vi "Fixated Autoadjust.vi"(10 "Input":variant, 11 "Data":T1) -> (2 "Fixated":bool, 3 "Adjustment":dbl[](array[numeric]))   [LabVIEW 2010]
uses:
  Core SubVIs/Controls/TYPE - Analog Data.ctl
  <vilib>/Analysis/baseanly.llb/Unimode.vi
  <vilib>/Analysis/NI_AALBase.lvlib
  Core SubVIs/Core SubVIs.lvlib
panel:
  out "Max. running window size":i32=1000
  in  "Learning rate":dbl=0.0003
  in  "Minimum for update":i32=40
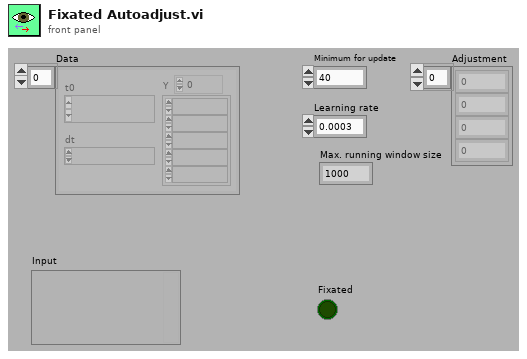
[diagram p1: front panel]
types:
  T1 = typedef "Core SubVIs.lvlib/TYPE - Analog Data.ctl" = waveform(dbl)[]
  T2 = cluster{"Trial Type":dbl, "Joystick Threshold":dbl, "Fixation Radius":dbl}
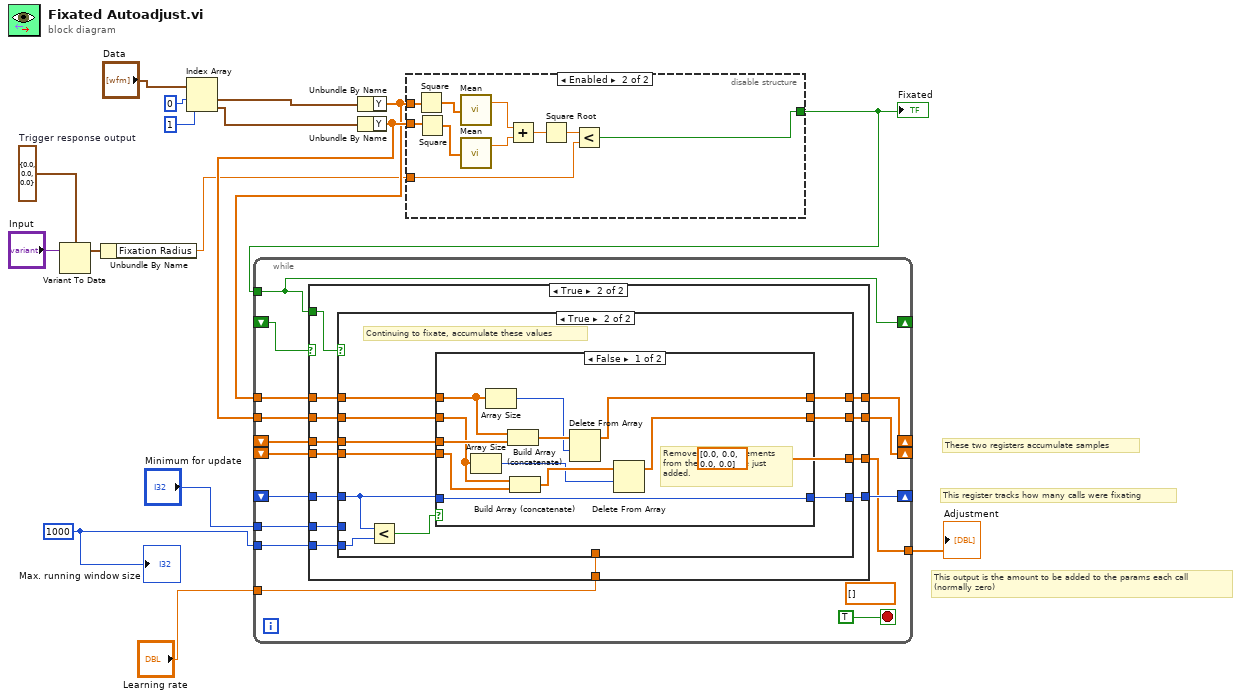
[diagram p0: block diagram]
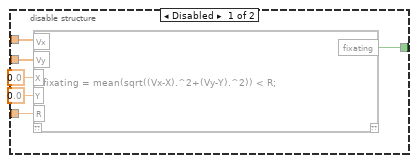
[diagram p2: hidden frame]
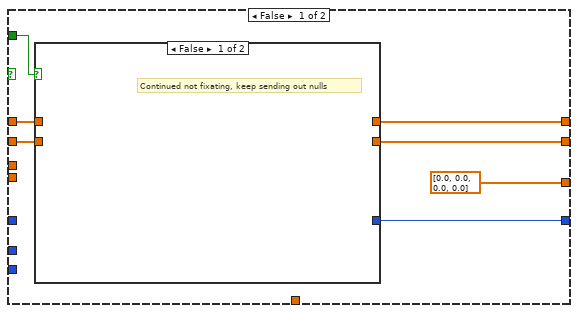
[diagram p3: hidden frame]
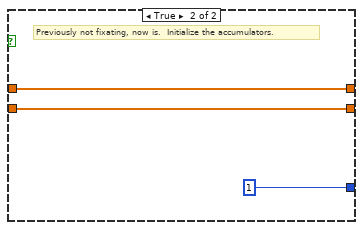
[diagram p4: hidden frame]
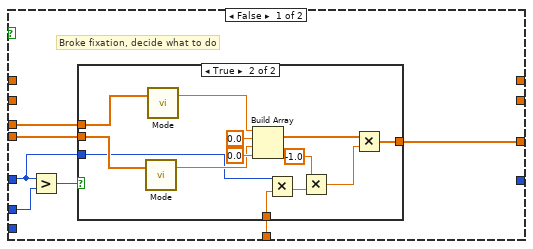
[diagram p5: hidden frame]
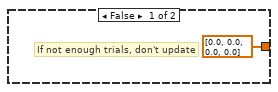
[diagram p6: hidden frame]
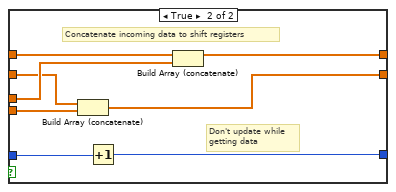
[diagram p7: hidden frame]
diagram:
  w3 = T2 {"Trial Type"=0.0, "Joystick Threshold"=0.0, "Fixation Radius"=0.0}  # Trigger response output
  w5 = 1000
  # "This output is the amount to be added to the params each call\n(normally zero)"
  # "These two registers accumulate samples"
  # "This register tracks how many calls were fixating"
  n1 = Variant To Data(Variant="Input", type=w3) -> (data=w2:T2)  [unwired: 1 in, 1 out]
  n2 = Unbundle By Name(w2) -> ("Fixation Radius"=w1:dbl)
  n3 = Index Array(array="Data", index #1=0 ("index"), index #2=1 ("index")) -> (element #1=w13:waveform(dbl), element #2=w12:waveform(dbl))
  n4 = Unbundle By Name(w13) -> ("Y"=w9:dbl[])
  n5 = Unbundle By Name(w12) -> ("Y"=w10:dbl[])
  n6 = disable-structure shown="Enabled" {
    disable-tunnel: w1 -> [w20 w24]
    disable-tunnel: [w19 w23] -> w11
    disable-tunnel: w10 -> [w18 w32]
    disable-tunnel: w9 -> [w17 w31]
    frame Disabled {
      n7 = mathscript code="fixating = mean(sqrt((Vx-X).^2+(Vy-Y).^2)) < R;"("Vx"=w17, "Vy"=w18, "X"=0.0, "Y"=0.0, "R"=w20) -> ("fixating"=w19:bool)  [unwired: 1 in, 1 out]
    }
    frame Enabled {
      n8 = Square(x=w31) -> (x^2=w29:dbl[])
      n9 = Square(x=w32) -> (x^2=w30:dbl[])
      n10 = call <vilib>:"Mean.vi"("X"=w29) -> ("mean"=w27:dbl)  [unwired: 1 out]
      n11 = call <vilib>:"Mean.vi"("X"=w30) -> ("mean"=w28:dbl)  [unwired: 1 out]
      n12 = Add(x=w27, y=w28) -> (x+y=w26:dbl)
      n13 = Square Root(x=w26) -> (sqrt(x)=w25:dbl)
      n14 = Less?(x=w25, y=w24) -> (x < y?=w23:bool)
    }
  }
  "Fixated" <- w11
  n15 = while {
    tunnel: w11 -> [w45]
    shift-right: [w45] -> _
    shift-left: _ -> [w46]
    shift-right: [w44] -> _
    shift-left: _ -> [w39]
    tunnel: w10 -> [w43]
    tunnel: w9 -> [w42]
    shift-right: [w34] -> _
    shift-left: _ -> [w41]
    shift-right: [w33] -> _
    shift-left: _ -> [w40]
    tunnel: "Minimum for update" -> [w38]
    tunnel: "Learning rate" -> [w37]
    tunnel: [w36] -> w6
    tunnel: w5 -> [w35]
    stop <- TRUE stop-if-true
    (unwired) dbl[] []
    n16 = case shown="True" w46 {
      tunnel: w45 -> [w54 w62]
      tunnel: [w53 w63] -> w44
      tunnel: w43 -> [w52 w66]
      tunnel: w42 -> [w51 w70]
      tunnel: [w50 w68] -> w34
      tunnel: [w49 w65] -> w33
      tunnel: w41 -> [_ w69]
      tunnel: w40 -> [_ w67]
      tunnel: w39 -> [_ w64]
      tunnel: w38 -> [_ w61]
      tunnel: w37 -> [_ w60]
      tunnel: [dbl[] [0.0, 0.0, 0.0, 0.0] w59] -> w36
      tunnel: w35 -> [_ w58]
      frame False {
        n17 = case shown="False" w54 {
          tunnel: [_ 1] -> w53
          tunnel: w52 -> [_ w55]
          tunnel: w51 -> [_ w56]
          tunnel: [_ w56] -> w50
          tunnel: [_ w55] -> w49
          frame False {
            # "Continued not fixating, keep sending out nulls"
          }
          frame True {
            # "Previously not fixating, now is.  Initialize the accumulators."
          }
        }
      }
      frame True {
        n18 = case shown="True" w62 {
          tunnel: w70 -> [_ w102]
          tunnel: w69 -> [w75 w101]
          tunnel: [_ w94] -> w68
          tunnel: w67 -> [w74 w100]
          tunnel: w66 -> [_ w99]
          tunnel: [_ w93] -> w65
          tunnel: w64 -> [w72 w92]
          tunnel: [_ w98] -> w63
          tunnel: w61 -> [w77 _]
          tunnel: w60 -> [w73 _]
          tunnel: [w71 dbl[] [0.0, 0.0, 0.0, 0.0]] -> w59
          tunnel: w58 -> [_ w96]
          frame False {
            # "Broke fixation, decide what to do"
            n19 = Greater?(x=w72, y=w77) -> (0:w76:bool)
            n20 = case shown="True" w76 {
              tunnel: w75 -> [_ w91]
              tunnel: w74 -> [_ w90]
              tunnel: w73 -> [_ w84]
              tunnel: w72 -> [_ w83]
              tunnel: [dbl[] [0.0, 0.0, 0.0, 0.0] w79] -> w71
              frame False {
                # "If not enough trials, don't update"
              }
              frame True {
                n21 = call-poly <vilib>:"Mode.vi"("X"=w90) -> ("mode"=w86:dbl)  [unwired: 1 in, 1 out]
                n22 = call-poly <vilib>:"Mode.vi"("X"=w91) -> ("mode"=w89:dbl)  [unwired: 1 in, 1 out]
                n23 = Build Array(w89, 0.0 ("element"), w86, 0.0 ("element")) -> (w85:dbl[])
                n24 = Multiply(x=w83, y=w84) -> (x*y=w82:dbl)
                n25 = Multiply(x=-1.0, y=w82) -> (x*y=w80:dbl)
                n26 = Multiply(x=w85, y=w80) -> (x*y=w79:dbl[])
              }
            }
          }
          frame True {
            # "Continuing to fixate, accumulate these values"
            n27 = Less?(x=w92, y=w96) -> (x < y?=w95:bool)
            n28 = case shown="False" w95 {
              tunnel: w102 -> [w111 w121]
              tunnel: w101 -> [w112 w120]
              tunnel: [w108 w119] -> w94
              tunnel: w100 -> [w107 w118]
              tunnel: w99 -> [w106 w117]
              tunnel: [w103 w116] -> w93
              tunnel: [w113 w115] -> w98
              tunnel: w92 -> [w113 w114]
              frame False {
                # "Remove as many elements\nfrom the array as we just\nadded."
                n29 = Array Size(array=w106) -> (size(s)=w104:i32)
                n30 = Array Size(array=w111) -> (size(s)=w109:i32)
                n31 = Build Array (concatenate)(w111, w112) -> (w110:dbl[])
                n32 = Build Array (concatenate)(w106, w107) -> (w105:dbl[])
                n33 = Delete From Array(array=w110, length=w109) -> (array with subset deleted=w108:dbl[])  [unwired: 1 in, 1 out]
                n34 = Delete From Array(array=w105, length=w104) -> (array with subset deleted=w103:dbl[])  [unwired: 1 in, 1 out]
              }
              frame True {
                # "Concatenate incoming data to shift registers"
                # "Don't update while\ngetting data"
                n35 = Build Array (concatenate)(w117, w118) -> (w116:dbl[])
                n36 = Increment(x=w114) -> (x+1=w115:i32)
                n37 = Build Array (concatenate)(w121, w120) -> (w119:dbl[])
              }
            }
          }
        }
      }
    }
  }
  "Adjustment" <- w6
  "Max. running window size" <- w5
